vi "data_waypoint_ref.vi"() -> ()   [LabVIEW 2019] (continued)
  out "way point part":cluster{"X":dbl, "Y":dbl}[](graph)=[{"X"=175275.58703968537, "Y"=530134.2259097229}, {"X"=175275.6113424378, "Y"=530134.2565077101}, {"X"=175275.63557628682, "Y"=530134.2880681476}, {"X"=175275.66020323776, "Y"=530134.3195641611}, {"X"=175275.68491628268, "Y"=530134.35081908}, {"X"=175275.7097711018, "Y"=530134.3817905674}, {"X"=175275.73389469017, "Y"=530134.4126088354}, {"X"=175275.7577146616, "Y"=530134.4423003837}, {"X"=175275.78100623479, "Y"=530134.4715351238}, {"X"=175275.80342291066, "Y"=530134.5005604674}, {"X"=175275.82593068006, "Y"=530134.5292381555}, {"X"=175275.84870407218, "Y"=530134.557576552}, {"X"=175275.8723047294, "Y"=530134.5861932964}, {"X"=175275.8962104465, "Y"=530134.6158257698}, {"X"=175275.9206685924, "Y"=530134.6465531515}, {"X"=175275.94534715984, "Y"=530134.6778314793}, {"X"=175275.97041945267, "Y"=530134.7092562574}, {"X"=175275.99540918533, "Y"=530134.7409198968}, {"X"=175276.0208479327, "Y"=530134.7722559111}, {"X"=175276.04626527152, "Y"=530134.8032423825}, {"X"=175276.0707201348, "Y"=530134.8340574529}, {"X"=175276.09469571977, "Y"=530134.8642524196}, {"X"=175276.11845871908, "Y"=530134.8938497994}, {"X"=175276.14216767476, "Y"=530134.9231443482}, {"X"=175276.16565515427, "Y"=530134.9527281164}, {"X"=175276.18933507518, "Y"=530134.9829883279}, {"X"=175276.21328929672, "Y"=530135.0137471656}, {"X"=175276.23786405282, "Y"=530135.0443687653}, {"X"=175276.26216325478, "Y"=530135.07556498}, {"X"=175276.28639760052, "Y"=530135.1066959022}, {"X"=175276.3104839446, "Y"=530135.1375020731}, {"X"=175276.33440064892, "Y"=530135.1675562614}, {"X"=175276.35738667226, "Y"=530135.1965088919}, {"X"=175276.37903969965, "Y"=530135.2246053237}, {"X"=175276.40010305776, "Y"=530135.2524926253}, {"X"=175276.42257118158, "Y"=530135.2821426697}, {"X"=175276.44697916886, "Y"=530135.3138823927}, {"X"=175276.47269765826, "Y"=530135.3469600595}, {"X"=175276.4987057177, "Y"=530135.3812077725}, {"X"=175276.52459011346, "Y"=530135.415572385}, {"X"=175276.54989015873, "Y"=530135.449730072}, {"X"=175276.57483091034, "Y"=530135.4828044904}, {"X"=175276.59904920924, "Y"=530135.5148000421}, {"X"=175276.62270533358, "Y"=530135.5457007147}, {"X"=175276.64582765175, "Y"=530135.5755130845}, {"X"=175276.66823122185, "Y"=530135.6040024065}, {"X"=175276.68969509072, "Y"=530135.6316354779}, {"X"=175276.71066645414, "Y"=530135.6586684603}, {"X"=175276.73236713343, "Y"=530135.6861043859}, {"X"=175276.75435481517, "Y"=530135.7147414407}, {"X"=175276.7766906527, "Y"=530135.7445894321}, {"X"=175276.79958941144, "Y"=530135.7757864564}, {"X"=175276.82353418818, "Y"=530135.8078460784}, {"X"=175276.8479998637, "Y"=530135.8408220143}, {"X"=175276.87281893456, "Y"=530135.874385132}, {"X"=175276.8982353833, "Y"=530135.9077689041}, {"X"=175276.92355676193, "Y"=530135.941353842}, {"X"=175276.94920471654, "Y"=530135.9748434767}, {"X"=175276.97503856523, "Y"=530136.0085911597}, {"X"=175277.00103956382, "Y"=530136.042549222}, {"X"=175277.0271864251, "Y"=530136.0773070601}, {"X"=175277.0538277369, "Y"=530136.1127238036}, {"X"=175277.08122741545, "Y"=530136.1490827955}, {"X"=175277.1097199428, "Y"=530136.1859668468}, {"X"=175277.13826682538, "Y"=530136.2235588295}, {"X"=175277.16623464657, "Y"=530136.2618339786}, {"X"=175277.19366071408, "Y"=530136.3005269243}, {"X"=175277.2211805134, "Y"=530136.3385669983}, {"X"=175277.24894896135, "Y"=530136.3759193327}, {"X"=175277.27651148668, "Y"=530136.4128305535}, {"X"=175277.30377007398, "Y"=530136.4488059506}, {"X"=175277.3310530873, "Y"=530136.4837557664}, {"X"=175277.35790209068, "Y"=530136.5187157434}, {"X"=175277.38489518996, "Y"=530136.5535776294}, {"X"=175277.41163428145, "Y"=530136.5885124052}, {"X"=175277.43827130183, "Y"=530136.6233775625}, {"X"=175277.4651897453, "Y"=530136.6581553189}, {"X"=175277.49179216905, "Y"=530136.6927042685}, {"X"=175277.5176344978, "Y"=530136.727524051}, {"X"=175277.54344339736, "Y"=530136.7624216232}, {"X"=175277.56908157616, "Y"=530136.7971010571}, {"X"=175277.59486848288, "Y"=530136.8314515362}, {"X"=175277.62049959434, "Y"=530136.8667358635}, {"X"=175277.6472220221, "Y"=530136.9020269552}, {"X"=175277.6753270872, "Y"=530136.9375892024}, {"X"=175277.70423989603, "Y"=530136.9740158635}, {"X"=175277.73315492744, "Y"=530137.0114946631}, {"X"=175277.762207521, "Y"=530137.0490629561}, {"X"=175277.79086273597, "Y"=530137.08704529}, {"X"=175277.81920082003, "Y"=530137.1247233516}, {"X"=175277.84718645428, "Y"=530137.1618353155}, {"X"=175277.87464469287, "Y"=530137.1979299895}, {"X"=175277.9008237915, "Y"=530137.2337065866}, {"X"=175277.9271261955, "Y"=530137.2689456482}, {"X"=175277.95360932988, "Y"=530137.3044938259}, {"X"=175277.98064951657, "Y"=530137.3403033918}, {"X"=175278.00823913375, "Y"=530137.376793897}, {"X"=175278.03589400547, "Y"=530137.4140821989}, {"X"=175278.06381256797, "Y"=530137.4518780371}, {"X"=175278.0928952896, "Y"=530137.4894506804}, {"X"=175278.12228673112, "Y"=530137.5271800106}, {"X"=175278.151430175, "Y"=530137.5652175064}, {"X"=175278.180067244, "Y"=530137.6036560485}, {"X"=175278.2089476153, "Y"=530137.6413968799}, {"X"=175278.23784769257, "Y"=530137.67891235}, {"X"=175278.26667870057, "Y"=530137.7167343476}, {"X"=175278.295506967, "Y"=530137.7548282683}, {"X"=175278.3247139495, "Y"=530137.7924860048}, {"X"=175278.35371856295, "Y"=530137.8306049308}, {"X"=175278.38247794105, "Y"=530137.8690675278}, {"X"=175278.41117485458, "Y"=530137.9076745918}, {"X"=175278.43986590861, "Y"=530137.9460974373}, {"X"=175278.46847093437, "Y"=530137.9841853591}, {"X"=175278.49675173132, "Y"=530138.0219634802}, {"X"=175278.52471101953, "Y"=530138.0600522002}, {"X"=175278.55337122487, "Y"=530138.097927977}, {"X"=175278.58284640842, "Y"=530138.1352219965}, {"X"=175278.61280407023, "Y"=530138.1730195764}, {"X"=175278.6421407967, "Y"=530138.212318413}, {"X"=175278.6718176569, "Y"=530138.2519125747}, {"X"=175278.70174630472, "Y"=530138.2918822337}, {"X"=175278.7324047895, "Y"=530138.33213164}, {"X"=175278.76330645662, "Y"=530138.3722427061}, {"X"=175278.7947664709, "Y"=530138.4115552426}, {"X"=175278.82585993598, "Y"=530138.4509254653}, {"X"=175278.85671998298, "Y"=530138.4901432156}, {"X"=175278.88660487908, "Y"=530138.5296956997}, {"X"=175278.91639916634, "Y"=530138.5691607723}, {"X"=175278.9459413744, "Y"=530138.6081526802}, {"X"=175278.97519875658, "Y"=530138.6466803991}, {"X"=175279.00399939533, "Y"=530138.6850196817}, {"X"=175279.0333091102, "Y"=530138.7223730155}, {"X"=175279.06206272755, "Y"=530138.760087587}, {"X"=175279.09082204034, "Y"=530138.7988298717}, {"X"=175279.12034452776, "Y"=530138.8386420244}, {"X"=175279.1511945661, "Y"=530138.8792682199}, {"X"=175279.18281582693, "Y"=530138.9203915691}, {"X"=175279.21403033624, "Y"=530138.9614550801}, {"X"=175279.2443611752, "Y"=530139.0023391879}, {"X"=175279.27433731925, "Y"=530139.0421966133}, {"X"=175279.30379101905, "Y"=530139.0806149871}, {"X"=175279.33186221574, "Y"=530139.1185080461}, {"X"=175279.35892676964, "Y"=530139.1559723445}, {"X"=175279.38686212158, "Y"=530139.1922598379}, {"X"=175279.41540915347, "Y"=530139.2284112311}, {"X"=175279.44399877635, "Y"=530139.2654858995}, {"X"=175279.47229163084, "Y"=530139.3037501057}, {"X"=175279.5011885739, "Y"=530139.3417073153}, {"X"=175279.5302888436, "Y"=530139.3795274108}, {"X"=175279.55929689365, "Y"=530139.4170148209}, {"X"=175279.58712148367, "Y"=530139.4547876343}, {"X"=175279.614104584, "Y"=530139.4922666025}, {"X"=175279.64106285188, "Y"=530139.5288355612}, {"X"=175279.66805218573, "Y"=530139.5639283156}, {"X"=175279.69406272576, "Y"=530139.5987243007}, {"X"=175279.72019882765, "Y"=530139.6337452154}, {"X"=175279.7465857226, "Y"=530139.6700028821}, {"X"=175279.77402264145, "Y"=530139.7072807357}, {"X"=175279.8023412458, "Y"=530139.7461663891}, {"X"=175279.83184920144, "Y"=530139.7864591549}, {"X"=175279.86223487387, "Y"=530139.8276150165}, {"X"=175279.89343681408, "Y"=530139.8689249574}, {"X"=175279.9246664868, "Y"=530139.910027272}, {"X"=175279.95597331063, "Y"=530139.9508596614}, {"X"=175279.98646708307, "Y"=530139.9914291999}, {"X"=175280.0165342933, "Y"=530140.0312308655}, {"X"=175280.0455922527, "Y"=530140.0703207663}, {"X"=175280.07421584064, "Y"=530140.1081000975}, {"X"=175280.10217132277, "Y"=530140.1449069497}, {"X"=175280.1291443291, "Y"=530140.1810696573}, {"X"=175280.15513247682, "Y"=530140.2166825664}, {"X"=175280.18117865722, "Y"=530140.2509501547}, {"X"=175280.206797209, "Y"=530140.2840913909}, {"X"=175280.23235000763, "Y"=530140.3165635753}, {"X"=175280.25719254743, "Y"=530140.350583895}, {"X"=175280.28322486824, "Y"=530140.3861567193}, {"X"=175280.31067604403, "Y"=530140.4234656083}, {"X"=175280.3394714572, "Y"=530140.4627371931}, {"X"=175280.36899300263, "Y"=530140.5034339112}, {"X"=175280.3984291721, "Y"=530140.5446147801}, {"X"=175280.42762195613, "Y"=530140.5855666273}, {"X"=175280.45709143404, "Y"=530140.6248306718}, {"X"=175280.48662985, "Y"=530140.6622443764}, {"X"=175280.51499879934, "Y"=530140.6989856332}, {"X"=175280.54198175855, "Y"=530140.7349207922}, {"X"=175280.56821058405, "Y"=530140.7692488853}, {"X"=175280.5935160324, "Y"=530140.8028483094}, {"X"=175280.61895653373, "Y"=530140.8353896387}, {"X"=175280.64395685605, "Y"=530140.8685493513}, {"X"=175280.66892636206, "Y"=530140.9029710654}, {"X"=175280.69431101237, "Y"=530140.9384925328}, {"X"=175280.72115648974, "Y"=530140.9743659461}, {"X"=175280.74851024564, "Y"=530141.0107827985}, {"X"=175280.77549811464, "Y"=530141.0483794013}, {"X"=175280.80221979975, "Y"=530141.0867248375}, {"X"=175280.83002676512, "Y"=530141.1242324503}, {"X"=175280.85869850015, "Y"=530141.1612214238}, {"X"=175280.88737895148, "Y"=530141.1984623082}, {"X"=175280.9154864763, "Y"=530141.2366638052}, {"X"=175280.94386501168, "Y"=530141.2751508438}, {"X"=175280.97276275096, "Y"=530141.3139804051}, {"X"=175281.00228102322, "Y"=530141.3529734996}, {"X"=175281.03115592728, "Y"=530141.3927687078}, {"X"=175281.0600630094, "Y"=530141.4329611481}, {"X"=175281.08951047983, "Y"=530141.4728734163}, {"X"=175281.1195389884, "Y"=530141.5124709872}, {"X"=175281.1496177038, "Y"=530141.5525733957}, {"X"=175281.1799730451, "Y"=530141.5930623271}, {"X"=175281.20985549872, "Y"=530141.6341930445}, {"X"=175281.24002660922, "Y"=530141.6758856092}, {"X"=175281.2701406386, "Y"=530141.7180455929}, {"X"=175281.30071187392, "Y"=530141.7596526246}, {"X"=175281.3314443854, "Y"=530141.8009806047}, {"X"=175281.36215111212, "Y"=530141.8419768134}, {"X"=175281.39229160105, "Y"=530141.8831999974}, {"X"=175281.42191398598, "Y"=530141.9244513493}, {"X"=175281.4515510467, "Y"=530141.9652731441}, {"X"=175281.48146043535, "Y"=530142.005928764}, {"X"=175281.51131504713, "Y"=530142.0472304844}, {"X"=175281.54193657986, "Y"=530142.088173672}, {"X"=175281.57268864528, "Y"=530142.1289266894}, {"X"=175281.60313783126, "Y"=530142.1699991305}, {"X"=175281.63309546496, "Y"=530142.2110941121}, {"X"=175281.66344358743, "Y"=530142.2512401207}, {"X"=175281.6938036245, "Y"=530142.2909221732}, {"X"=175281.7242871103, "Y"=530142.3298147498}, {"X"=175281.75410497762, "Y"=530142.3688757736}, {"X"=175281.78380300084, "Y"=530142.4081480255}, {"X"=175281.8133516878, "Y"=530142.4481421259}, {"X"=175281.843129746, "Y"=530142.4887193365}, {"X"=175281.87290404478, "Y"=530142.530421954}, {"X"=175281.9035498242, "Y"=530142.5720776024}, {"X"=175281.93428441955, "Y"=530142.6138128963}, {"X"=175281.96503678558, "Y"=530142.6558666679}, {"X"=175281.9955543286, "Y"=530142.697891169}, {"X"=175282.02619666213, "Y"=530142.7392804611}, {"X"=175282.05613426614, "Y"=530142.7804920393}, {"X"=175282.085671532, "Y"=530142.8211187952}, {"X"=175282.11518036062, "Y"=530142.8620131105}, {"X"=175282.1456811949, "Y"=530142.9028811874}, {"X"=175282.1771792938, "Y"=530142.9437019224}, {"X"=175282.20884129676, "Y"=530142.9851325951}, {"X"=175282.2397414916, "Y"=530143.0274545162}, {"X"=175282.27097983484, "Y"=530143.0694003062}, {"X"=175282.30222752306, "Y"=530143.1112106664}, {"X"=175282.33341880344, "Y"=530143.1525184269}, {"X"=175282.36387121098, "Y"=530143.1931857627}, {"X"=175282.39415697358, "Y"=530143.2332143132}, {"X"=175282.42362074467, "Y"=530143.273250842}, {"X"=175282.4527898988, "Y"=530143.313107335}, {"X"=175282.48128543983, "Y"=530143.3534241924}, {"X"=175282.51088211057, "Y"=530143.3931717661}, {"X"=175282.54090583324, "Y"=530143.4323542686}, {"X"=175282.5705854428, "Y"=530143.471693168}, {"X"=175282.59956877265, "Y"=530143.5110152598}, {"X"=175282.6287490361, "Y"=530143.5495365605}, {"X"=175282.6578151003, "Y"=530143.588080396}, {"X"=175282.68706937856, "Y"=530143.626769067}, {"X"=175282.7166015784, "Y"=530143.6659829883}, {"X"=175282.7467854581, "Y"=530143.7057077412}, {"X"=175282.7773134472, "Y"=530143.7458743079}, {"X"=175282.80814411398, "Y"=530143.7859523029}, {"X"=175282.838184342, "Y"=530143.826524301}, {"X"=175282.8683331907, "Y"=530143.8669838827}, {"X"=175282.89893667438, "Y"=530143.906620824}, {"X"=175282.9292553414, "Y"=530143.9460954601}, {"X"=175282.95864972533, "Y"=530143.9860345288}, {"X"=175282.98848236992, "Y"=530144.0253041666}, {"X"=175283.0181754902, "Y"=530144.0647196089}, {"X"=175283.04813967334, "Y"=530144.1041386905}, {"X"=175283.0777535639, "Y"=530144.1434200734}, {"X"=175283.10767498845, "Y"=530144.1824585982}, {"X"=175283.13729311575, "Y"=530144.2216767089}, {"X"=175283.16682575422, "Y"=530144.2604411386}, {"X"=175283.19558793583, "Y"=530144.298968117}, {"X"=175283.2241672666, "Y"=530144.3373668897}, {"X"=175283.25312463212, "Y"=530144.3756990653}, {"X"=175283.2826412646, "Y"=530144.4144435665}, {"X"=175283.31204253566, "Y"=530144.4543149145}, {"X"=175283.3421730828, "Y"=530144.4945792174}, {"X"=175283.3722977522, "Y"=530144.5352508556}, {"X"=175283.40277253534, "Y"=530144.5759991499}, {"X"=175283.4329718328, "Y"=530144.6164463753}, {"X"=175283.46352714679, "Y"=530144.6565706909}, {"X"=175283.49419215746, "Y"=530144.6963472951}, {"X"=175283.52462383907, "Y"=530144.7353998523}, {"X"=175283.55396090678, "Y"=530144.7748296679}, {"X"=175283.5835840078, "Y"=530144.8145316618}, {"X"=175283.61356165347, "Y"=530144.8549118419}, {"X"=175283.64420085354, "Y"=530144.8958449971}, {"X"=175283.6745753304, "Y"=530144.9374226541}, {"X"=175283.7054805737, "Y"=530144.9784593498}, {"X"=175283.73611770716, "Y"=530145.0195933951}, {"X"=175283.76646929348, "Y"=530145.060618409}, {"X"=175283.79638575143, "Y"=530145.1009754644}, {"X"=175283.82613484285, "Y"=530145.1407492278}, {"X"=175283.85577592644, "Y"=530145.1808429519}, {"X"=175283.885663239, "Y"=530145.2218282747}, {"X"=175283.91601352586, "Y"=530145.2642128682}, {"X"=175283.947973915, "Y"=530145.3071054613}, {"X"=175283.98073738883, "Y"=530145.3501865757}, {"X"=175284.0130592979, "Y"=530145.3937184858}, {"X"=175284.04495574543, "Y"=530145.4371550977}, {"X"=175284.07744431793, "Y"=530145.4792348221}, {"X"=175284.10977979988, "Y"=530145.5207656174}, {"X"=175284.14209092426, "Y"=530145.5618481026}, {"X"=175284.1734844176, "Y"=530145.6035470525}, {"X"=175284.20526964756, "Y"=530145.64591853}, {"X"=175284.23726074316, "Y"=530145.6887122538}, {"X"=175284.26911709429, "Y"=530145.7317705223}, {"X"=175284.3002081578, "Y"=530145.7757400281}, {"X"=175284.3324970653, "Y"=530145.8188969061}, {"X"=175284.3652071701, "Y"=530145.861604157}, {"X"=175284.39764851984, "Y"=530145.9041912265}, {"X"=175284.42918119673, "Y"=530145.9465290459}, {"X"=175284.46056710478, "Y"=530145.9883589816}, {"X"=175284.49216892465, "Y"=530146.0298153689}, {"X"=175284.52417019266, "Y"=530146.0712561457}, {"X"=175284.55620185586, "Y"=530146.1139909273}, {"X"=175284.58914297097, "Y"=530146.1578373206}, {"X"=175284.62234006467, "Y"=530146.2022778434}, {"X"=175284.65546114062, "Y"=530146.246771863}, {"X"=175284.6880941868, "Y"=530146.290381658}, {"X"=175284.7208188328, "Y"=530146.3323175148}, {"X"=175284.75239886277, "Y"=530146.3738938312}, {"X"=175284.7831501817, "Y"=530146.4147045729}, {"X"=175284.8133402377, "Y"=530146.4547267567}, {"X"=175284.84401715046, "Y"=530146.4940394099}, {"X"=175284.87397091367, "Y"=530146.5335351082}, {"X"=175284.9036312302, "Y"=530146.5732458769}, {"X"=175284.93309855444, "Y"=530146.613594275}, {"X"=175284.96356257205, "Y"=530146.6534025557}, {"X"=175284.99386236374, "Y"=530146.6933911182}, {"X"=175285.02346019607, "Y"=530146.7338401279}, {"X"=175285.05236272336, "Y"=530146.7740026298}, {"X"=175285.08160787256, "Y"=530146.8135059732}, {"X"=175285.11075855847, "Y"=530146.8522171556}, {"X"=175285.1397029091, "Y"=530146.8900477202}, {"X"=175285.16758823174, "Y"=530146.9277071673}, {"X"=175285.1958097519, "Y"=530146.9649305547}, {"X"=175285.22430324028, "Y"=530147.0021642376}, {"X"=175285.25292049572, "Y"=530147.0399147498}, {"X"=175285.2813211958, "Y"=530147.0781209449}, {"X"=175285.31057523662, "Y"=530147.1161381598}, {"X"=175285.34005196817, "Y"=530147.1539760306}, {"X"=175285.36896240644, "Y"=530147.1923216721}, {"X"=175285.39717128137, "Y"=530147.2306616167}, {"X"=175285.42578933577, "Y"=530147.2680836085}, {"X"=175285.45344861108, "Y"=530147.3059856722}, {"X"=175285.48089067373, "Y"=530147.3438228995}, {"X"=175285.5080579749, "Y"=530147.3816032234}, {"X"=175285.5362745623, "Y"=530147.4192572538}, {"X"=175285.56450088962, "Y"=530147.457507248}, {"X"=175285.59262162892, "Y"=530147.4962980582}, {"X"=175285.62062185156, "Y"=530147.535671899}, {"X"=175285.64955586256, "Y"=530147.5747999209}, {"X"=175285.67873101955, "Y"=530147.6137008192}, {"X"=175285.70778441665, "Y"=530147.6521647931}, {"X"=175285.73595734, "Y"=530147.6906291493}, {"X"=175285.76424656826, "Y"=530147.7282851851}, {"X"=175285.79254815428, "Y"=530147.7653274323}, {"X"=175285.82039661068, "Y"=530147.8022034307}, {"X"=175285.8475120278, "Y"=530147.8389140045}, {"X"=175285.87503700587, "Y"=530147.8754358034}, {"X"=175285.90290258938, "Y"=530147.9124127475}, {"X"=175285.9312492372, "Y"=530147.9503150036}, {"X"=175285.96021217544, "Y"=530147.9893430532}, {"X"=175285.99025259638, "Y"=530148.0293912095}, {"X"=175286.020547502, "Y"=530148.0707260491}, {"X"=175286.0507198295, "Y"=530148.1125473701}, {"X"=175286.0801991385, "Y"=530148.1548557479}, {"X"=175286.11029842027, "Y"=530148.1962377818}, {"X"=175286.140521968, "Y"=530148.236507368}, {"X"=175286.1702336265, "Y"=530148.2765109926}, {"X"=175286.19897639108, "Y"=530148.3165685348}, {"X"=175286.22822459688, "Y"=530148.3559109423}, {"X"=175286.25734444545, "Y"=530148.3955811377}, {"X"=175286.28666392548, "Y"=530148.4356613915}, {"X"=175286.31565993704, "Y"=530148.4762897632}, {"X"=175286.3452906467, "Y"=530148.5167775253}, {"X"=175286.37519197192, "Y"=530148.5571168768}, {"X"=175286.4050008174, "Y"=530148.5970369751}, {"X"=175286.43396749627, "Y"=530148.6376310271}, {"X"=175286.46322490054, "Y"=530148.6782874814}, {"X"=175286.492849835, "Y"=530148.7186198815}, {"X"=175286.52249772992, "Y"=530148.7589289073}, {"X"=175286.55175465223, "Y"=530148.7991236621}, {"X"=175286.58125565466, "Y"=530148.8385840784}, {"X"=175286.61029576242, "Y"=530148.8779481912}, {"X"=175286.63886234077, "Y"=530148.9171383454}, {"X"=175286.6662366717, "Y"=530148.9560379102}, {"X"=175286.69313776202, "Y"=530148.994561523}, {"X"=175286.71988594692, "Y"=530149.0322998049}, {"X"=175286.74621013305, "Y"=530149.0686387003}, {"X"=175286.77196082624, "Y"=530149.105147988}, {"X"=175286.79863885418, "Y"=530149.142826546}, {"X"=175286.826449198, "Y"=530149.1826948401}, {"X"=175286.85571812605, "Y"=530149.22455435}, {"X"=175286.8856057402, "Y"=530149.2680490734}, {"X"=175286.9166891728, "Y"=530149.3112439304}, {"X"=175286.94756222956, "Y"=530149.3539899159}, {"X"=175286.97788231372, "Y"=530149.3960549736}, {"X"=175287.0072642036, "Y"=530149.4374746449}, {"X"=175287.036659181, "Y"=530149.4776268187}, {"X"=175287.06515292102, "Y"=530149.5170491512}, {"X"=175287.09290277224, "Y"=530149.5556312968}, {"X"=175287.119605925, "Y"=530149.5949179686}, {"X"=175287.14739103278, "Y"=530149.6343412843}, {"X"=175287.17584614863, "Y"=530149.6735817129}, {"X"=175287.2043462658, "Y"=530149.713065068}, {"X"=175287.23238548372, "Y"=530149.7533488837}, {"X"=175287.2611683341, "Y"=530149.7940866544}, {"X"=175287.29022015305, "Y"=530149.8350178539}, {"X"=175287.31949523537, "Y"=530149.8762647061}, {"X"=175287.3483993774, "Y"=530149.9178800166}, {"X"=175287.37800341408, "Y"=530149.9598373151}, {"X"=175287.40788540026, "Y"=530150.0026284064}, {"X"=175287.43796715222, "Y"=530150.0458750587}, {"X"=175287.46768028973, "Y"=530150.0890806267}, {"X"=175287.4980408877, "Y"=530150.131969081}, {"X"=175287.52849568735, "Y"=530150.1743611491}, {"X"=175287.55858161338, "Y"=530150.2166244559}, {"X"=175287.587891292, "Y"=530150.2584882879}, {"X"=175287.61718485222, "Y"=530150.299393249}, {"X"=175287.6459290996, "Y"=530150.3402576577}, {"X"=175287.6745216954, "Y"=530150.3816607958}, {"X"=175287.70312189191, "Y"=530150.4232381617}, {"X"=175287.73260160128, "Y"=530150.4650881741}, {"X"=175287.76249647667, "Y"=530150.5074463824}, {"X"=175287.79194968793, "Y"=530150.5502209846}, {"X"=175287.82063771554, "Y"=530150.5936437859}, {"X"=175287.85010417973, "Y"=530150.6364072509}, {"X"=175287.8799999824, "Y"=530150.6784802239}, {"X"=175287.90960605638, "Y"=530150.7208281889}, {"X"=175287.93873272298, "Y"=530150.7643085173}, {"X"=175287.96876992864, "Y"=530150.8083710499}, {"X"=175287.99941347007, "Y"=530150.8537847098}, {"X"=175288.03114061506, "Y"=530150.8995947163}, {"X"=175288.06276278125, "Y"=530150.9458489771}, {"X"=175288.09491236706, "Y"=530150.9922304217}, {"X"=175288.12711197292, "Y"=530151.0378525751}, {"X"=175288.15885105054, "Y"=530151.0829045124}, {"X"=175288.18957201828, "Y"=530151.1275432631}, {"X"=175288.22029953293, "Y"=530151.1716992052}, {"X"=175288.25093068994, "Y"=530151.2162216855}, {"X"=175288.28194385857, "Y"=530151.2608229464}, {"X"=175288.31247756336, "Y"=530151.3053401643}, {"X"=175288.3432649797, "Y"=530151.3499842685}, {"X"=175288.37381855643, "Y"=530151.3946312824}, {"X"=175288.40417486875, "Y"=530151.4390691165}, {"X"=175288.43387214167, "Y"=530151.4838041204}, {"X"=175288.4640216559, "Y"=530151.5281038334}, {"X"=175288.49419391077, "Y"=530151.5723058113}, {"X"=175288.52442907562, "Y"=530151.6168139238}, {"X"=175288.5542325439, "Y"=530151.6615153196}, {"X"=175288.58497125428, "Y"=530151.7061640078}, {"X"=175288.6160333851, "Y"=530151.7508494728}, {"X"=175288.6471765447, "Y"=530151.7953782111}, {"X"=175288.67735389853, "Y"=530151.8404070201}, {"X"=175288.7079524178, "Y"=530151.8849762128}, {"X"=175288.73890247892, "Y"=530151.928907307}, {"X"=175288.76994925848, "Y"=530151.9731943812}, {"X"=175288.80061505685, "Y"=530152.0180497186}, {"X"=175288.8317122577, "Y"=530152.0632134323}, {"X"=175288.86321392213, "Y"=530152.1088598475}, {"X"=175288.89513094307, "Y"=530152.1541798481}, {"X"=175288.92626476596, "Y"=530152.1997463321}, {"X"=175288.95799837503, "Y"=530152.2447483455}, {"X"=175288.98898292525, "Y"=530152.2889612439}, {"X"=175289.01901433212, "Y"=530152.3328628676}, {"X"=175289.04869555627, "Y"=530152.376364868}, {"X"=175289.07902414582, "Y"=530152.419217908}, {"X"=175289.10912839917, "Y"=530152.4628917961}, {"X"=175289.13898367598, "Y"=530152.50744099}, {"X"=175289.16920329822, "Y"=530152.5520878835}, {"X"=175289.200499284, "Y"=530152.5967771014}, {"X"=175289.23222510127, "Y"=530152.6409434144}, {"X"=175289.26360565764, "Y"=530152.6851751207}, {"X"=175289.29417483156, "Y"=530152.7294092241}, {"X"=175289.32498934455, "Y"=530152.7727347375}, {"X"=175289.35533826269, "Y"=530152.8164722754}, {"X"=175289.385890799, "Y"=530152.8604711375}, {"X"=175289.41661120942, "Y"=530152.904625996}, {"X"=175289.4478910891, "Y"=530152.9495616502}, {"X"=175289.47917020373, "Y"=530152.9951376967}, {"X"=175289.5106185431, "Y"=530153.0407265619}, {"X"=175289.54200313758, "Y"=530153.08602594}, {"X"=175289.5739645148, "Y"=530153.130472353}, {"X"=175289.60522496788, "Y"=530153.1748287205}, {"X"=175289.6366590831, "Y"=530153.2192023303}, {"X"=175289.6678968938, "Y"=530153.2639904988}, {"X"=175289.69931618578, "Y"=530153.3099423731}, {"X"=175289.73108270628, "Y"=530153.3561928844}, {"X"=175289.76287250203, "Y"=530153.402526566}, {"X"=175289.7944634813, "Y"=530153.4493247548}, {"X"=175289.82722049116, "Y"=530153.4953348278}, {"X"=175289.8601326513, "Y"=530153.5407928433}, {"X"=175289.89234136775, "Y"=530153.5862074348}, {"X"=175289.9231350958, "Y"=530153.6320945667}, {"X"=175289.95472487184, "Y"=530153.6784854437}, {"X"=175289.98763897427, "Y"=530153.7249001521}, {"X"=175290.0213877559, "Y"=530153.7711048503}, {"X"=175290.05441688612, "Y"=530153.8180774795}, {"X"=175290.0870279125, "Y"=530153.865045794}, {"X"=175290.1190894426, "Y"=530153.9119114052}, {"X"=175290.15082290868, "Y"=530153.9583695601}, {"X"=175290.18253651966, "Y"=530154.004402696}, {"X"=175290.215824471, "Y"=530154.0499339624}, {"X"=175290.24876343764, "Y"=530154.0957714727}, {"X"=175290.28090772417, "Y"=530154.1421662602}, {"X"=175290.31260737777, "Y"=530154.1888720124}, {"X"=175290.34510314872, "Y"=530154.2349083878}, {"X"=175290.37745346018, "Y"=530154.2805800489}, {"X"=175290.40967781737, "Y"=530154.3255950455}, {"X"=175290.4415173953, "Y"=530154.3698930992}, {"X"=175290.47334424395, "Y"=530154.4146795312}, {"X"=175290.50540644318, "Y"=530154.4602743543}, {"X"=175290.5380738031, "Y"=530154.5068251977}, {"X"=175290.57155401353, "Y"=530154.5544701797}, {"X"=175290.60687618723, "Y"=530154.6022528902}, {"X"=175290.64227715097, "Y"=530154.6503194917}, {"X"=175290.6771000642, "Y"=530154.6985121064}, {"X"=175290.71074572636, "Y"=530154.7463930005}, {"X"=175290.74366782108, "Y"=530154.7937166628}, {"X"=175290.77674741115, "Y"=530154.8397823889}, {"X"=175290.8104922183, "Y"=530154.8852446075}, {"X"=175290.84345047412, "Y"=530154.9319166768}, {"X"=175290.8771305831, "Y"=530154.9791648488}, {"X"=175290.91168912026, "Y"=530155.0269198505}, {"X"=175290.94661003543, "Y"=530155.0750045214}, {"X"=175290.981122192, "Y"=530155.1229516666}, {"X"=175291.01579159318, "Y"=530155.1701547412}, {"X"=175291.04955919375, "Y"=530155.2164370784}, {"X"=175291.08231414267, "Y"=530155.262653598}, {"X"=175291.11492730505, "Y"=530155.3085508951}, {"X"=175291.14872001382, "Y"=530155.3537377286}, {"X"=175291.182644366, "Y"=530155.3991095183}, {"X"=175291.21636701853, "Y"=530155.4442699214}, {"X"=175291.24936465317, "Y"=530155.4895811882}, {"X"=175291.28248111415, "Y"=530155.5349365}, {"X"=175291.31537208255, "Y"=530155.580122668}, {"X"=175291.348325878, "Y"=530155.6252864538}, {"X"=175291.38153227052, "Y"=530155.6705005467}, {"X"=175291.41516056712, "Y"=530155.7158055122}, {"X"=175291.44858402072, "Y"=530155.7616338248}, {"X"=175291.48274548614, "Y"=530155.8069127973}, {"X"=175291.51713847913, "Y"=530155.8517049672}, {"X"=175291.55134679007, "Y"=530155.8960504106}, {"X"=175291.58456519523, "Y"=530155.9396351947}, {"X"=175291.61696642355, "Y"=530155.9821591497}, {"X"=175291.6479902135, "Y"=530156.023771541}, {"X"=175291.6785537982, "Y"=530156.0649235916}, {"X"=175291.70969666803, "Y"=530156.1063669323}, {"X"=175291.7420121854, "Y"=530156.1480631868}, {"X"=175291.77421945485, "Y"=530156.1905977037}, {"X"=175291.80641845273, "Y"=530156.2342298953}, {"X"=175291.83880961206, "Y"=530156.2778426528}, {"X"=175291.8714862793, "Y"=530156.3212525729}, {"X"=175291.903615614, "Y"=530156.3652911794}, {"X"=175291.9363788722, "Y"=530156.4089272545}, {"X"=175291.9693198524, "Y"=530156.4530544727}, {"X"=175292.00263982284, "Y"=530156.4980373809}, {"X"=175292.03573972572, "Y"=530156.5440875158}, {"X"=175292.06968311957, "Y"=530156.5908099515}, {"X"=175292.10416577995, "Y"=530156.6374730819}, {"X"=175292.13854745447, "Y"=530156.6838335177}, {"X"=175292.1720661163, "Y"=530156.7301088271}, {"X"=175292.2050774269, "Y"=530156.7758551223}, {"X"=175292.23774666685, "Y"=530156.8212483841}, {"X"=175292.2703950841, "Y"=530156.8658914415}, {"X"=175292.30284617713, "Y"=530156.9103042324}, {"X"=175292.33573019976, "Y"=530156.9552418168}, {"X"=175292.3690841089, "Y"=530157.0006197365}, {"X"=175292.40287209605, "Y"=530157.0463115734}, {"X"=175292.43625491866, "Y"=530157.0924818472}, {"X"=175292.46991898818, "Y"=530157.1379065764}, {"X"=175292.50292587615, "Y"=530157.1830557807}, {"X"=175292.53606117488, "Y"=530157.2272967426}, {"X"=175292.56777705185, "Y"=530157.2717072674}, {"X"=175292.59928240773, "Y"=530157.317118397}, {"X"=175292.63191829307, "Y"=530157.3626160842}, {"X"=175292.66587593383, "Y"=530157.4075682566}, {"X"=175292.69985293486, "Y"=530157.4527767475}, {"X"=175292.73331970134, "Y"=530157.49827975}, {"X"=175292.76675738787, "Y"=530157.5444332153}, {"X"=175292.8009040642, "Y"=530157.5910063332}, {"X"=175292.8354354053, "Y"=530157.637958995}, {"X"=175292.87064782495, "Y"=530157.6854778919}, {"X"=175292.90666329346, "Y"=530157.7325748918}, {"X"=175292.94218916725, "Y"=530157.7803559012}, {"X"=175292.97651543948, "Y"=530157.8283546561}, {"X"=175293.01087843996, "Y"=530157.8758927135}, {"X"=175293.04497236086, "Y"=530157.9235003758}, {"X"=175293.07881658027, "Y"=530157.9705383087}, {"X"=175293.11260566092, "Y"=530158.0172023829}, {"X"=175293.14703717566, "Y"=530158.0636470264}, {"X"=175293.1813700373, "Y"=530158.1105791891}, {"X"=175293.21539555187, "Y"=530158.1584179054}, {"X"=175293.2495375595, "Y"=530158.205812335}, {"X"=175293.28470608912, "Y"=530158.252269229}, {"X"=175293.3199063943, "Y"=530158.2983886322}, {"X"=175293.35488698122, "Y"=530158.3438949328}, {"X"=175293.3886446154, "Y"=530158.389809945}, {"X"=175293.4223983855, "Y"=530158.4359169754}, {"X"=175293.45635716093, "Y"=530158.4824551338}, {"X"=175293.49104767398, "Y"=530158.5290177691}, {"X"=175293.52591940033, "Y"=530158.5751547926}, {"X"=175293.56061870293, "Y"=530158.6210958796}, {"X"=175293.59411550115, "Y"=530158.6668718222}, {"X"=175293.6271809516, "Y"=530158.7120597042}, {"X"=175293.65945930034, "Y"=530158.7576716585}, {"X"=175293.69267942, "Y"=530158.8030433188}, {"X"=175293.72706808845, "Y"=530158.8484792291}, {"X"=175293.76185547217, "Y"=530158.895451116}, {"X"=175293.7965144529, "Y"=530158.9433356876}, {"X"=175293.83203452808, "Y"=530158.9915551107}, {"X"=175293.86796527763, "Y"=530159.0399619979}, {"X"=175293.90361325, "Y"=530159.0885983519}, {"X"=175293.93887625565, "Y"=530159.1373534874}, {"X"=175293.97487363513, "Y"=530159.1852274456}, {"X"=175294.01073365632, "Y"=530159.2333814944}, {"X"=175294.04643691002, "Y"=530159.2821408798}, {"X"=175294.0818756446, "Y"=530159.3307123703}, {"X"=175294.11788264144, "Y"=530159.3791445598}, {"X"=175294.15405635608, "Y"=530159.4270401951}, {"X"=175294.19031250803, "Y"=530159.474657012}, {"X"=175294.2255617339, "Y"=530159.5217474012}, {"X"=175294.25969315338, "Y"=530159.5685591893}, {"X"=175294.29275883175, "Y"=530159.6156260639}, {"X"=175294.32651326683, "Y"=530159.6616609548}, {"X"=175294.3607518941, "Y"=530159.7075834295}, {"X"=175294.3953102612, "Y"=530159.754094294}, {"X"=175294.4301660572, "Y"=530159.800839571}, {"X"=175294.46538930168, "Y"=530159.8478312608}, {"X"=175294.5005892464, "Y"=530159.8944334593}, {"X"=175294.5360717114, "Y"=530159.9401191891}, {"X"=175294.57088286872, "Y"=530159.9855471951}, {"X"=175294.60512637242, "Y"=530160.0307227217}, {"X"=175294.63868134032, "Y"=530160.0764041571}, {"X"=175294.67373468378, "Y"=530160.1216560913}, {"X"=175294.7093190078, "Y"=530160.167040749}, {"X"=175294.74458629126, "Y"=530160.2136494077}, {"X"=175294.7794420138, "Y"=530160.2609707027}, {"X"=175294.81483305173, "Y"=530160.3092915086}, {"X"=175294.85090509735, "Y"=530160.3593561125}, {"X"=175294.88806120938, "Y"=530160.4102709948}, {"X"=175294.92585483048, "Y"=530160.4622982909}, {"X"=175294.96463635506, "Y"=530160.5147089018}, {"X"=175295.00314084318, "Y"=530160.5674932406}, {"X"=175295.04201721685, "Y"=530160.6190278914}, {"X"=175295.08002002342, "Y"=530160.6696039869}, {"X"=175295.1164572531, "Y"=530160.7191503169}, {"X"=175295.15120238528, "Y"=530160.7677160925}, {"X"=175295.18513989958, "Y"=530160.8154596288}, {"X"=175295.21911985, "Y"=530160.8622751979}, {"X"=175295.25361585215, "Y"=530160.908367834}, {"X"=175295.2882631498, "Y"=530160.9541026478}, {"X"=175295.3227068247, "Y"=530160.9995739195}, {"X"=175295.35650395526, "Y"=530161.0453733961}, {"X"=175295.39054459677, "Y"=530161.090246534}, {"X"=175295.4242712038, "Y"=530161.1346622286}, {"X"=175295.45741238436, "Y"=530161.1797045011}, {"X"=175295.49052893237, "Y"=530161.2251053321}, {"X"=175295.52422381577, "Y"=530161.2716753556}, {"X"=175295.5584969615, "Y"=530161.3190916035}, {"X"=175295.59356381797, "Y"=530161.3671225884}, {"X"=175295.62898613833, "Y"=530161.4158406355}, {"X"=175295.66490363725, "Y"=530161.4645672088}, {"X"=175295.70087106727, "Y"=530161.5140039441}, {"X"=175295.7368334574, "Y"=530161.563833585}, {"X"=175295.77286787695, "Y"=530161.6140581218}, {"X"=175295.80940447663, "Y"=530161.6645608615}, {"X"=175295.84631290415, "Y"=530161.7143954771}, {"X"=175295.88293148752, "Y"=530161.7641654665}, {"X"=175295.91866648968, "Y"=530161.8137837979}, {"X"=175295.95399056026, "Y"=530161.862829545}, {"X"=175295.9882959008, "Y"=530161.9112501208}, {"X"=175296.021704602, "Y"=530161.9589974427}, {"X"=175296.05467506434, "Y"=530162.0062210971}, {"X"=175296.08883693878, "Y"=530162.0522559017}, {"X"=175296.12335942886, "Y"=530162.0980232735}, {"X"=175296.15767913012, "Y"=530162.1438101135}, {"X"=175296.19184323237, "Y"=530162.18969841}, {"X"=175296.22616491732, "Y"=530162.2364574812}, {"X"=175296.26090724123, "Y"=530162.2837780067}, {"X"=175296.29650390253, "Y"=530162.3312458408}, {"X"=175296.33225156722, "Y"=530162.3800550482}, {"X"=175296.36839006183, "Y"=530162.4298308986}, {"X"=175296.40405752033, "Y"=530162.4808744899}, {"X"=175296.4404195736, "Y"=530162.5316652008}, {"X"=175296.4771856306, "Y"=530162.5818831403}, {"X"=175296.5143190418, "Y"=530162.6314185419}, {"X"=175296.55121999886, "Y"=530162.6796261277}, {"X"=175296.58696759774, "Y"=530162.7272156009}, {"X"=175296.62106253332, "Y"=530162.7745791067}, {"X"=175296.65513370547, "Y"=530162.8216951848}, {"X"=175296.6894842066, "Y"=530162.8689147633}, {"X"=175296.7245051825, "Y"=530162.9161112749}, {"X"=175296.7594826378, "Y"=530162.9641680548}, {"X"=175296.7949428259, "Y"=530163.0125164114}, {"X"=175296.83066872833, "Y"=530163.0611569866}, {"X"=175296.8668875833, "Y"=530163.1102511483}, {"X"=175296.90347265196, "Y"=530163.1594751914}, {"X"=175296.94033878695, "Y"=530163.2096906174}, {"X"=175296.97742890092, "Y"=530163.2601628694}, {"X"=175297.0145870955, "Y"=530163.3102930847}, {"X"=175297.0517672564, "Y"=530163.3603633035}, {"X"=175297.0892145761, "Y"=530163.4100154234}, {"X"=175297.1260384531, "Y"=530163.4594196689}, {"X"=175297.16179432158, "Y"=530163.5083098755}, {"X"=175297.1968335202, "Y"=530163.5568792308}, {"X"=175297.2321241116, "Y"=530163.6047908057}, {"X"=175297.26783519427, "Y"=530163.6517155846}, {"X"=175297.3031716078, "Y"=530163.6989466816}, {"X"=175297.3376430369, "Y"=530163.7460238435}, {"X"=175297.37241788793, "Y"=530163.7935651409}, {"X"=175297.40764496886, "Y"=530163.8421672372}, {"X"=175297.44412403886, "Y"=530163.8908943782}, {"X"=175297.4814756149, "Y"=530163.9405212577}, {"X"=175297.51936847973, "Y"=530163.9910710508}, {"X"=175297.5573672983, "Y"=530164.0433064074}, {"X"=175297.595877763, "Y"=530164.0960252604}, {"X"=175297.63482324645, "Y"=530164.1484764633}, {"X"=175297.67408375622, "Y"=530164.201420622}, {"X"=175297.71312810254, "Y"=530164.2540568792}, {"X"=175297.7516670672, "Y"=530164.3059288258}, {"X"=175297.78913671337, "Y"=530164.3565442422}, {"X"=175297.82573620637, "Y"=530164.4067560205}, {"X"=175297.8615577048, "Y"=530164.4559778853}, {"X"=175297.8972371134, "Y"=530164.5047762007}, {"X"=175297.93302551022, "Y"=530164.553887177}, {"X"=175297.96961301554, "Y"=530164.6033398478}, {"X"=175298.00658313325, "Y"=530164.653376285}, {"X"=175298.04413234367, "Y"=530164.7030403184}, {"X"=175298.08174063195, "Y"=530164.7529128302}, {"X"=175298.11949670635, "Y"=530164.8033376161}, {"X"=175298.15754264174, "Y"=530164.8535340244}, {"X"=175298.19573262517, "Y"=530164.9039153553}, {"X"=175298.2333517534, "Y"=530164.9547600736}, {"X"=175298.2709253971, "Y"=530165.0063984748}, {"X"=175298.30921058325, "Y"=530165.0575242384}, {"X"=175298.34725989297, "Y"=530165.108563021}, {"X"=175298.3849848592, "Y"=530165.160152141}, {"X"=175298.42313040857, "Y"=530165.2113859762}, {"X"=175298.46161175598, "Y"=530165.2629473361}, {"X"=175298.5006422235, "Y"=530165.3141863251}, {"X"=175298.53957860355, "Y"=530165.3662590976}, {"X"=175298.57924604914, "Y"=530165.4196282434}, {"X"=175298.61979824462, "Y"=530165.4744453614}, {"X"=175298.66179051698, "Y"=530165.5306877274}, {"X"=175298.70499840498, "Y"=530165.5885357952}, {"X"=175298.74955290352, "Y"=530165.6482533285}, {"X"=175298.79480152024, "Y"=530165.7087545921}, {"X"=175298.83997422215, "Y"=530165.7702460737}, {"X"=175298.8847225618, "Y"=530165.8314136203}, {"X"=175298.9291021474, "Y"=530165.8912926009}, {"X"=175298.97281817885, "Y"=530165.9496397171}, {"X"=175299.01543963805, "Y"=530166.0068768775}, {"X"=175299.05688362545, "Y"=530166.0634271845}, {"X"=175299.09825262203, "Y"=530166.1191808339}, {"X"=175299.13975714424, "Y"=530166.173434664}, {"X"=175299.18070865513, "Y"=530166.2269953544}, {"X"=175299.22062828136, "Y"=530166.2793770946}, {"X"=175299.25974002617, "Y"=530166.3308455878}, {"X"=175299.297952328, "Y"=530166.3812912287}, {"X"=175299.33612488734, "Y"=530166.4305771838}, {"X"=175299.37402761978, "Y"=530166.4784788326}, {"X"=175299.41189246927, "Y"=530166.5255504185}, {"X"=175299.44854593184, "Y"=530166.5730484385}, {"X"=175299.48464680242, "Y"=530166.620295045}, {"X"=175299.5206186963, "Y"=530166.667360014}, {"X"=175299.5570817157, "Y"=530166.7139596118}, {"X"=175299.59393444148, "Y"=530166.760246189}, {"X"=175299.63101704643, "Y"=530166.8075875615}, {"X"=175299.66873832993, "Y"=530166.8558371342}, {"X"=175299.70755977381, "Y"=530166.9049891003}, {"X"=175299.74702618556, "Y"=530166.954779551}, {"X"=175299.78702946118, "Y"=530167.0048947148}, {"X"=175299.8269780119, "Y"=530167.0550766316}, {"X"=175299.86691015412, "Y"=530167.1045016735}, {"X"=175299.9056200963, "Y"=530167.1539902581}, {"X"=175299.94444108658, "Y"=530167.202690514}, {"X"=175299.9832469312, "Y"=530167.2507615263}, {"X"=175300.02239172766, "Y"=530167.2984286564}, {"X"=175300.06160983795, "Y"=530167.3454263278}, {"X"=175300.10023907598, "Y"=530167.3924845605}, {"X"=175300.13795698716, "Y"=530167.4389938845}, {"X"=175300.17463229306, "Y"=530167.4854940797}, {"X"=175300.21027157555, "Y"=530167.53151233}, {"X"=175300.2456148467, "Y"=530167.5762784209}, {"X"=175300.28083256615, "Y"=530167.6208229107}, {"X"=175300.31683014592, "Y"=530167.6648911891}, {"X"=175300.35295156413, "Y"=530167.7092010507}, {"X"=175300.38885968522, "Y"=530167.754471571}, {"X"=175300.42531408952, "Y"=530167.7996572366}, {"X"=175300.4626722015, "Y"=530167.8446127126}, {"X"=175300.49978768127, "Y"=530167.8895922136}, {"X"=175300.5366776678, "Y"=530167.9350018955}, {"X"=175300.57296706524, "Y"=530167.9810026871}, {"X"=175300.60997343756, "Y"=530168.02653078}, {"X"=175300.64725950157, "Y"=530168.0722844577}, {"X"=175300.6848355032, "Y"=530168.1178341768}, {"X"=175300.72194708392, "Y"=530168.1629945957}, {"X"=175300.75843372697, "Y"=530168.2077007085}, {"X"=175300.79459920572, "Y"=530168.2516353095}, {"X"=175300.8309390622, "Y"=530168.2958279934}, {"X"=175300.86721646803, "Y"=530168.3407689049}, {"X"=175300.9041467231, "Y"=530168.3860186503}, {"X"=175300.94086441226, "Y"=530168.431876116}, {"X"=175300.97748970473, "Y"=530168.4773398549}, {"X"=175301.01311529457, "Y"=530168.5226245311}, {"X"=175301.04880451673, "Y"=530168.5675605212}, {"X"=175301.08470138145, "Y"=530168.6111218947}, {"X"=175301.11998015357, "Y"=530168.6544464744}, {"X"=175301.1544579749, "Y"=530168.6983050416}, {"X"=175301.1899404005, "Y"=530168.7422039253}, {"X"=175301.2262133977, "Y"=530168.787153732}, {"X"=175301.26329977365, "Y"=530168.8327792599}, {"X"=175301.30040072044, "Y"=530168.8794402435}, {"X"=175301.33783310797, "Y"=530168.9261524099}, {"X"=175301.37482062684, "Y"=530168.9724974196}, {"X"=175301.41083388752, "Y"=530169.0185789398}, {"X"=175301.44611475465, "Y"=530169.0635150287}, {"X"=175301.48104166967, 
